vi "Calibration - Slope Trigger (eFGV).vi"(7 "Action":T2, 8 "error in":errorcluster, 11 "Calib":T1={"Timeout"=-1, "LC MC"=[], "TD MC"=[], "Motor Pulse"=0, "Disp M"=[], "LC Unit"=[], "Disp Unit"=[], "TD Unit"=[], "LC Name"=[], "TD Name"=[], "Machine"=enum."Please Select", "Sensor Port"=[]}) -> (0 "error out":errorcluster, 2 "Calib ref":refnum<user-event>, 3 "Calib out":T1={"Timeout"=-1, "LC MC"=[], "TD MC"=[], "Motor Pulse"=0, "Disp M"=[], "LC Unit"=[], "Disp Unit"=[], "TD Unit"=[], "LC Name"=[], "TD Name"=[], "Machine"=enum."Please Select", "Sensor Port"=[]})   [LabVIEW 2019]
uses:
  Controls/eFGV States.ctl
  Controls/Calibration - Data Structure.ctl
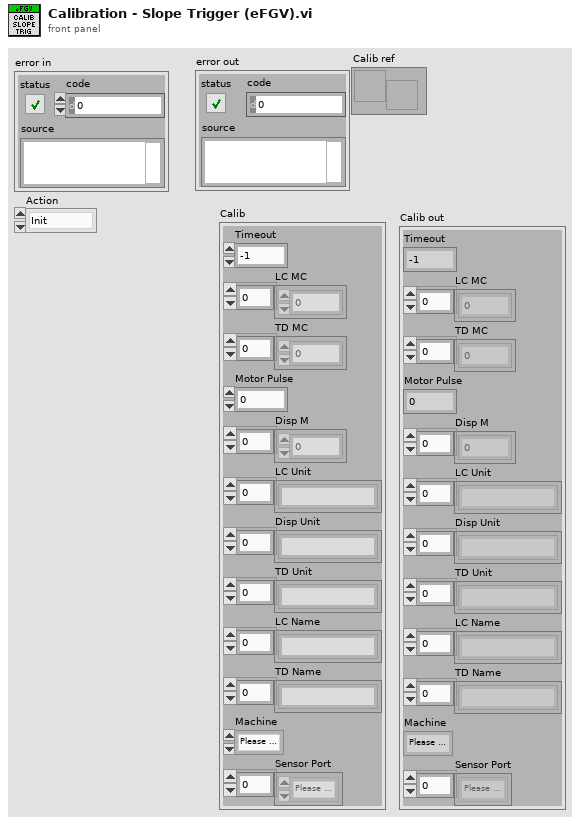
[diagram p1: front panel]
types:
  T1 = typedef "Calibration - Data Structure.ctl" = cluster{"Timeout":i32, "LC MC":dbl[], "TD MC":dbl[], "Motor Pulse":u64, "Disp M":dbl[], "LC Unit":string[], "Disp Unit":string[], "TD Unit":string[], "LC Name":string[], "TD Name":string[], "Machine":enum16{"Please Select", "Motor 1", "Motor 2", "Motor 3", "Motor 4", "Motor 5", "Motor 6", "Motor 7", "Motor 8", "Motor 9"}, "Sensor Port":enum16{"Please Select", "LC 1", "LC 2", "LC 3", "LC 4", "LC 5", "LC 6", "LC 7", "LC 8", "TD 1", "TD 2", "TD 3", "TD 4", "TD 5", "TD 6", "TD 7", "TD 8", "TD 9", "TD 10", "TD 11", "TD 12"}[]}
  T2 = typedef "eFGV States.ctl" = enum16{"Init", "Read", "Write", "Exit"}
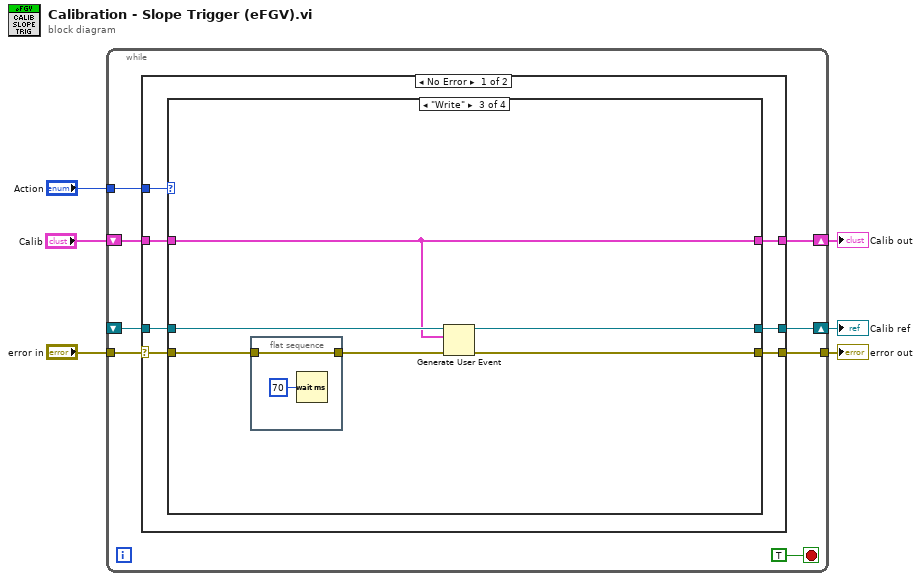
[diagram p0: block diagram]
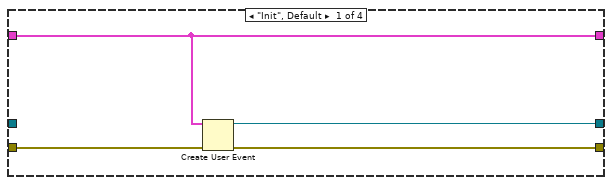
[diagram p2: hidden frame]
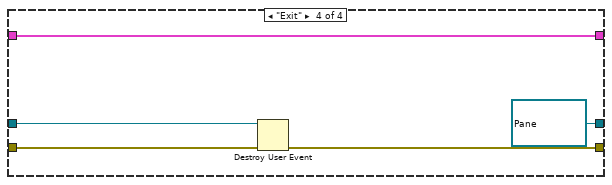
[diagram p4: hidden frame]
diagram:
  n1 = while {
    tunnel: "error in" -> [w13]
    tunnel: [w12] -> w5
    tunnel: "Action" -> [w11]
    shift-right: [w9] -> w2
    shift-left: "Calib" -> [w10]
    shift-right: [w8] -> w1
    shift-left: _ -> [w7]
    stop <- TRUE stop-if-true
    n2 = case shown="No Error" w13 {
      selector: w13 -> [w20 w44]
      tunnel: [w21 w44] -> w12
      tunnel: w11 -> [w19 _]
      tunnel: w10 -> [w18 w43]
      tunnel: [w17 w43] -> w9
      tunnel: w7 -> [w16 w42]
      tunnel: [w15 w42] -> w8
      frame No Error {
        n3 = case shown="\"Write\"" w19 {
          tunnel: [w24 w28 w34 w41] -> w21
          tunnel: w20 -> [w25 w28 w30 w40]
          tunnel: w18 -> [w23 w27 w32 w38]
          tunnel: [w23 w27 w32 w38] -> w17
          tunnel: w16 -> [_ w26 w33 w39]
          tunnel: [w22 w26 w31 refnum<user-event> refnum ("Calib")] -> w15
          frame "Init", Default {
            n4 = Create User Event(user event datatype=w23, error in=w25) -> (user event=w22:refnum<user-event>, error out=w24:errorcluster)
          }
          frame "Read" {
          }
          frame "Write" {
            n5 = flat-sequence {
              tunnel: [w35] -> w29
              tunnel: w30 -> [w35]
              frame #0 {
                n6 = Wait (ms)(milliseconds to wait=u32 70) -> ()  [unwired: 1 out]
              }
            }
            n7 = Generate User Event(user event=w33, event data cluster=w32, error in=w29) -> (user event out=w31:refnum<user-event>, error out=w34:errorcluster)  [unwired: 1 in]
          }
          frame "Exit" {
            n8 = Destroy User Event(user event=w39, error in=w40) -> (error out=w41:errorcluster)
          }
        }
      }
      frame Error {
      }
    }
  }
  "error out" <- w5
  "Calib out" <- w2
  "Calib ref" <- w1
